vi "Automatic Execution On Power On.vi"(4 "error in (no error)":errorcluster, 5 "Number of times of execution":i32=1 min=1 max=2000000000, 6 "Program Number":i32=1 min=1 max=100, 7 "VISA resource name":refnum<visa-resource-name>) -> (0 "error out":errorcluster, 3 "VISA resource name out":refnum<visa-resource-name>)   [LabVIEW 2019, in "Newport ESP301.lvlib"]
doc: "Sets the program number that is automatically executed on power on."
uses:
  Newport ESP301.lvlib
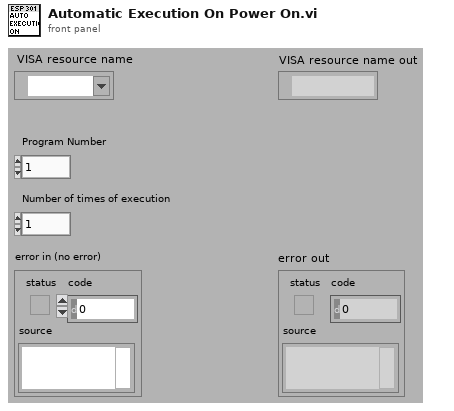
[diagram p1: front panel]
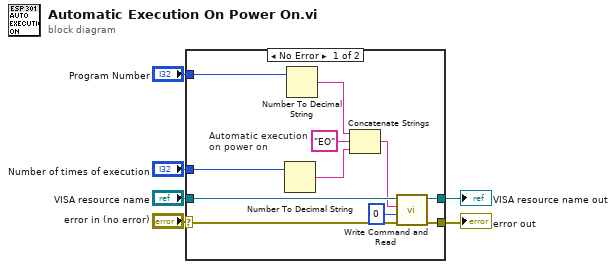
[diagram p0: block diagram]
diagram:
  n1 = case shown="No Error" "error in (no error)" {
    selector: "error in (no error)" -> [w14 w19]
    tunnel: [w16 w19] -> w6
    tunnel: "VISA resource name" -> [w17 w18]
    tunnel: [w15 w18] -> w5
    tunnel: "Program Number" -> [w10 _]
    tunnel: "Number of times of execution" -> [w8 _]
    frame No Error {
      w13 = "EO"  # Automatic execution on power on
      n2 = Number To Decimal String(number=w8) -> (decimal integer string=w7:string)  [unwired: 1 in]
      n3 = Number To Decimal String(number=w10) -> (decimal integer string=w12:string)  [unwired: 1 in]
      n4 = Concatenate Strings(w12, w13, w7) -> (w11:string)
      n5 = call "Write Command and Read.vi"("error in (no error)"=w14, "Bytes to read (100)"=u32 0, "Command"=w11, "VISA resource name"=w17) -> ("error out"=w16:errorcluster, "VISA resource name out"=w15:refnum<visa-resource-name>)  [unwired: 3 in, 1 out]
    }
    frame Error {
    }
  }
  "error out" <- w6
  "VISA resource name out" <- w5
